vi "checkemail.vi"(11 "email":string) -> (0 "valid email":bool, 1 "last three letters":string, 2 "institution":string, 3 "local":string)   [LabVIEW 2015, in "AguaClara Library.lvlib"]
uses:
  AguaClara Library.lvlib
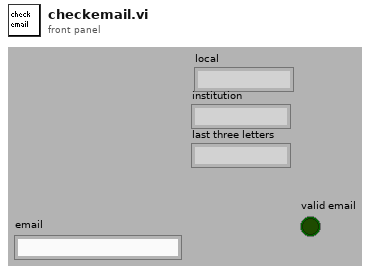
[diagram p1: front panel]
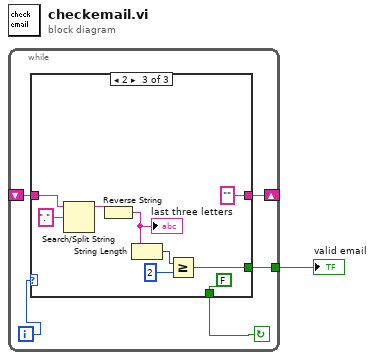
[diagram p0: block diagram]
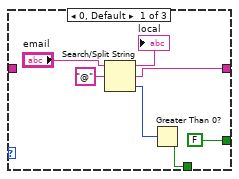
[diagram p2: hidden frame]
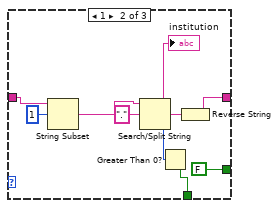
[diagram p3: hidden frame]
diagram:
  n1 = while {
    shift-right: [w6] -> _
    shift-left: _ -> [w3]
    tunnel: [w2] -> w1
    i -> [w4]
    stop <- w5 continue-if-true
    n2 = case shown="2" w4 {
      tunnel: [w11 w18 "" ("email")] -> w6
      tunnel: [w8 w17 FALSE] -> w5
      tunnel: w3 -> [_ w19 w27]
      tunnel: [FALSE FALSE w26] -> w2
      frame 0, Default {
        n3 = Search/Split String(string="email", search string/char (-)="@") -> (substring before match=→"local":string, match + rest of string=w11:string, offset of match=w9:i32)  [unwired: 1 in]
        n4 = Greater Than 0?(x=w9) -> (x > 0?=w8:bool)
      }
      frame 1 {
        n5 = String Subset(string=w19, offset (0)=1) -> (substring=w22:string)  [unwired: 1 in]
        n6 = Search/Split String(string=w22, search string/char (-)=".") -> (substring before match=→"institution":string, match + rest of string=w23:string, offset of match=w14:i32)  [unwired: 1 in]
        n7 = Greater Than 0?(x=w14) -> (x > 0?=w17:bool)
        n8 = Reverse String(1:w23) -> (0:w18:string)
      }
      frame 2 {
        n9 = Search/Split String(string=w27, search string/char (-)=".") -> (substring before match=w29:string)  [unwired: 1 in, 2 out]
        n10 = Reverse String(1:w29) -> (0:w30:string)
        "last three letters" <- w30
        n11 = String Length(string=w30) -> (length=w31:i32)
        n12 = Greater Or Equal?(x=w31, y=2) -> (x >= y?=w26:bool)
      }
    }
  }
  "valid email" <- w1
